vi "Init.vi"(8 "error in (no error)":errorcluster, 9 "Poll interval":i32, 10 "Message type":refnum<class "BaseMessage.lvclass">, 11 "BaseDriver in":refnum<class "BaseDriver.lvclass">) -> (0 "error out":errorcluster, 1 "Message queue":T1, 3 "BaseDriver out":refnum<class "BaseDriver.lvclass">)   [LabVIEW 2013, in "BaseDriver.lvclass"]
doc: "Initializes queues in a new driver. Wire the default type of message to \"Message type\""
uses:
  BaseDriver.lvclass
  message_queue.ctl
  Message/BaseMessage/BaseMessage.lvclass
  BaseDriver.lvclass/BaseDriver.ctl
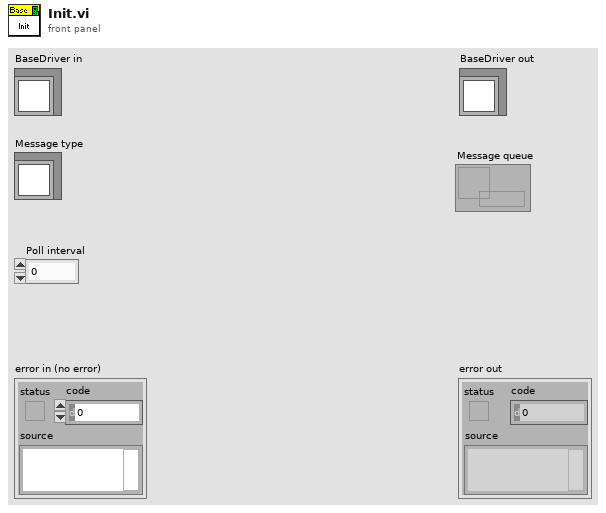
[diagram p1: front panel]
types:
  T1 = typedef "message_queue.ctl" = refnum<queue>
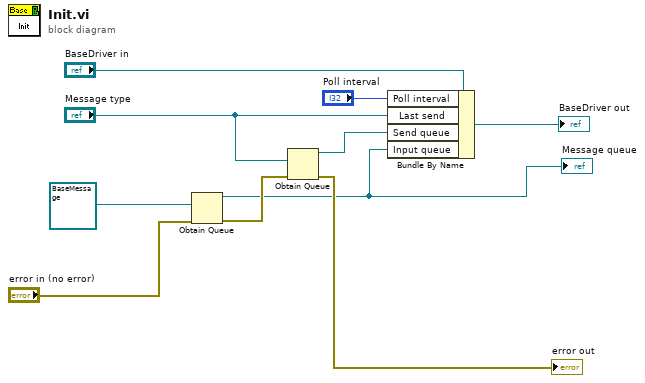
[diagram p0: block diagram]
diagram:
  n1 = Obtain Queue(element data type=refnum<class "BaseMessage.lvclass"> refnum ("Message type 2"), error in (no error)="error in (no error)") -> (queue out=w3:refnum<queue>, error out=w4:errorcluster)  [unwired: 3 in, 1 out]
  "Message queue" <- w3
  n2 = Obtain Queue(element data type="Message type", error in (no error)=w4) -> (queue out=w8:refnum<queue>, error out=→"error out":errorcluster)  [unwired: 3 in, 1 out]
  n3 = Bundle By Name(cluster="BaseDriver in", "Poll interval"="Poll interval", "Last send"="Message type", "Send queue"=w8, "Input queue"=w3) -> (→"BaseDriver out":refnum<class "BaseDriver.lvclass">)
